vi "Simple Read.vi"(4 "Boolean in":refnum<class "Abs_Boolean.lvclass">) -> (1 "Boolean":bool)   [LabVIEW 2021, in "Abs_Boolean.lvclass"]
uses:
  Abs_Boolean.lvclass
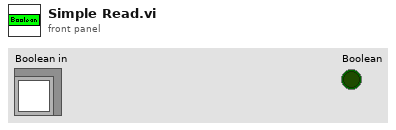
[diagram p1: front panel]
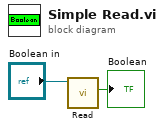
[diagram p0: block diagram]
diagram:
  n1 = call-dynamic "Read.vi"("Boolean in"="Boolean in") -> ("Boolean"=→"Boolean":bool)  [unwired: 8 in, 2 out]
